vi "nii_head.vi"(8 "error in (no error)":errorcluster, 11 "file (use dialog)":path) -> (0 "error out":errorcluster, 3 "Data":T1 {"slice orientation" items=["transverse unflipped", "coronal unflipped", "sagittal unflipped", "transverse flipped", "coronal flipped", "sagittal flipped"]}, 4 "non-flip":bool, 5 "head":u8[](array[numeric]) format="%.0x")   [LabVIEW 2014]
uses:
  control/head_data.ctl
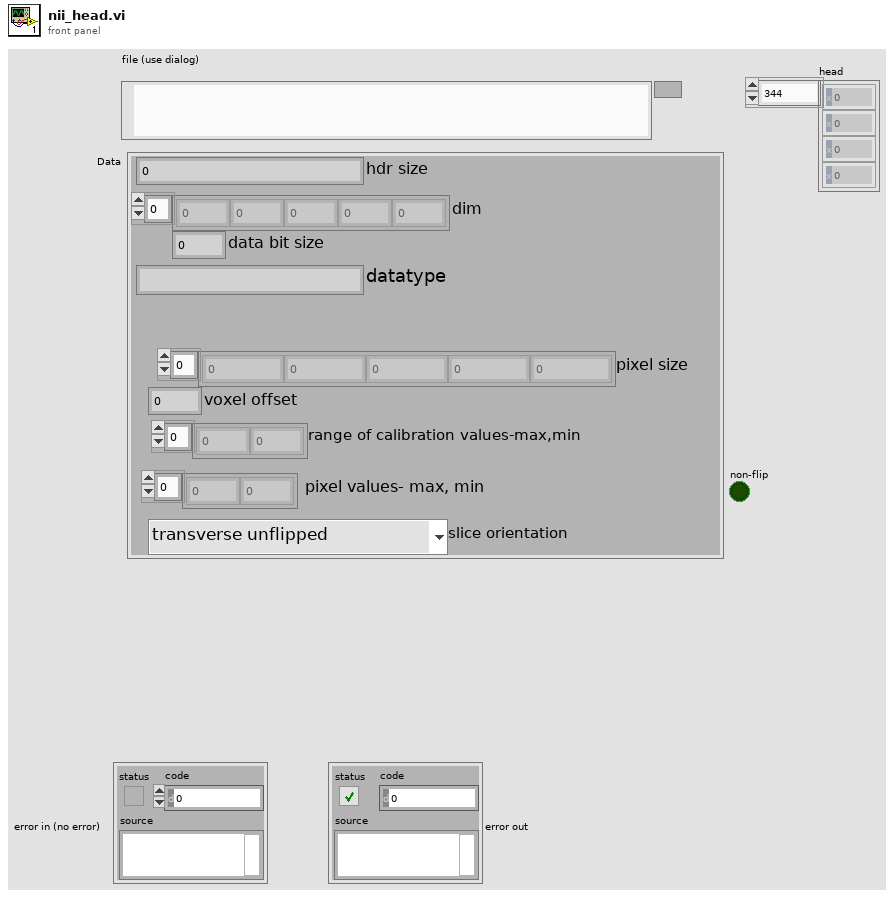
[diagram p1: front panel]
types:
  T1 = typedef "head_data.ctl" = cluster{"hdr size":i32, "dim":i32[], "data bit size":i32, "datatype":string, "pixel size ":sgl[], "voxel offset":sgl, "range of calibration values-max,min":sgl[], " pixel values- max, min":sgl[], "slice orientation":u16}
  T2 = enum16{"u_int8", "int8", "u_int16", "int16", "u_int32", "int32", "u_int64", "int64", "float", "double"}
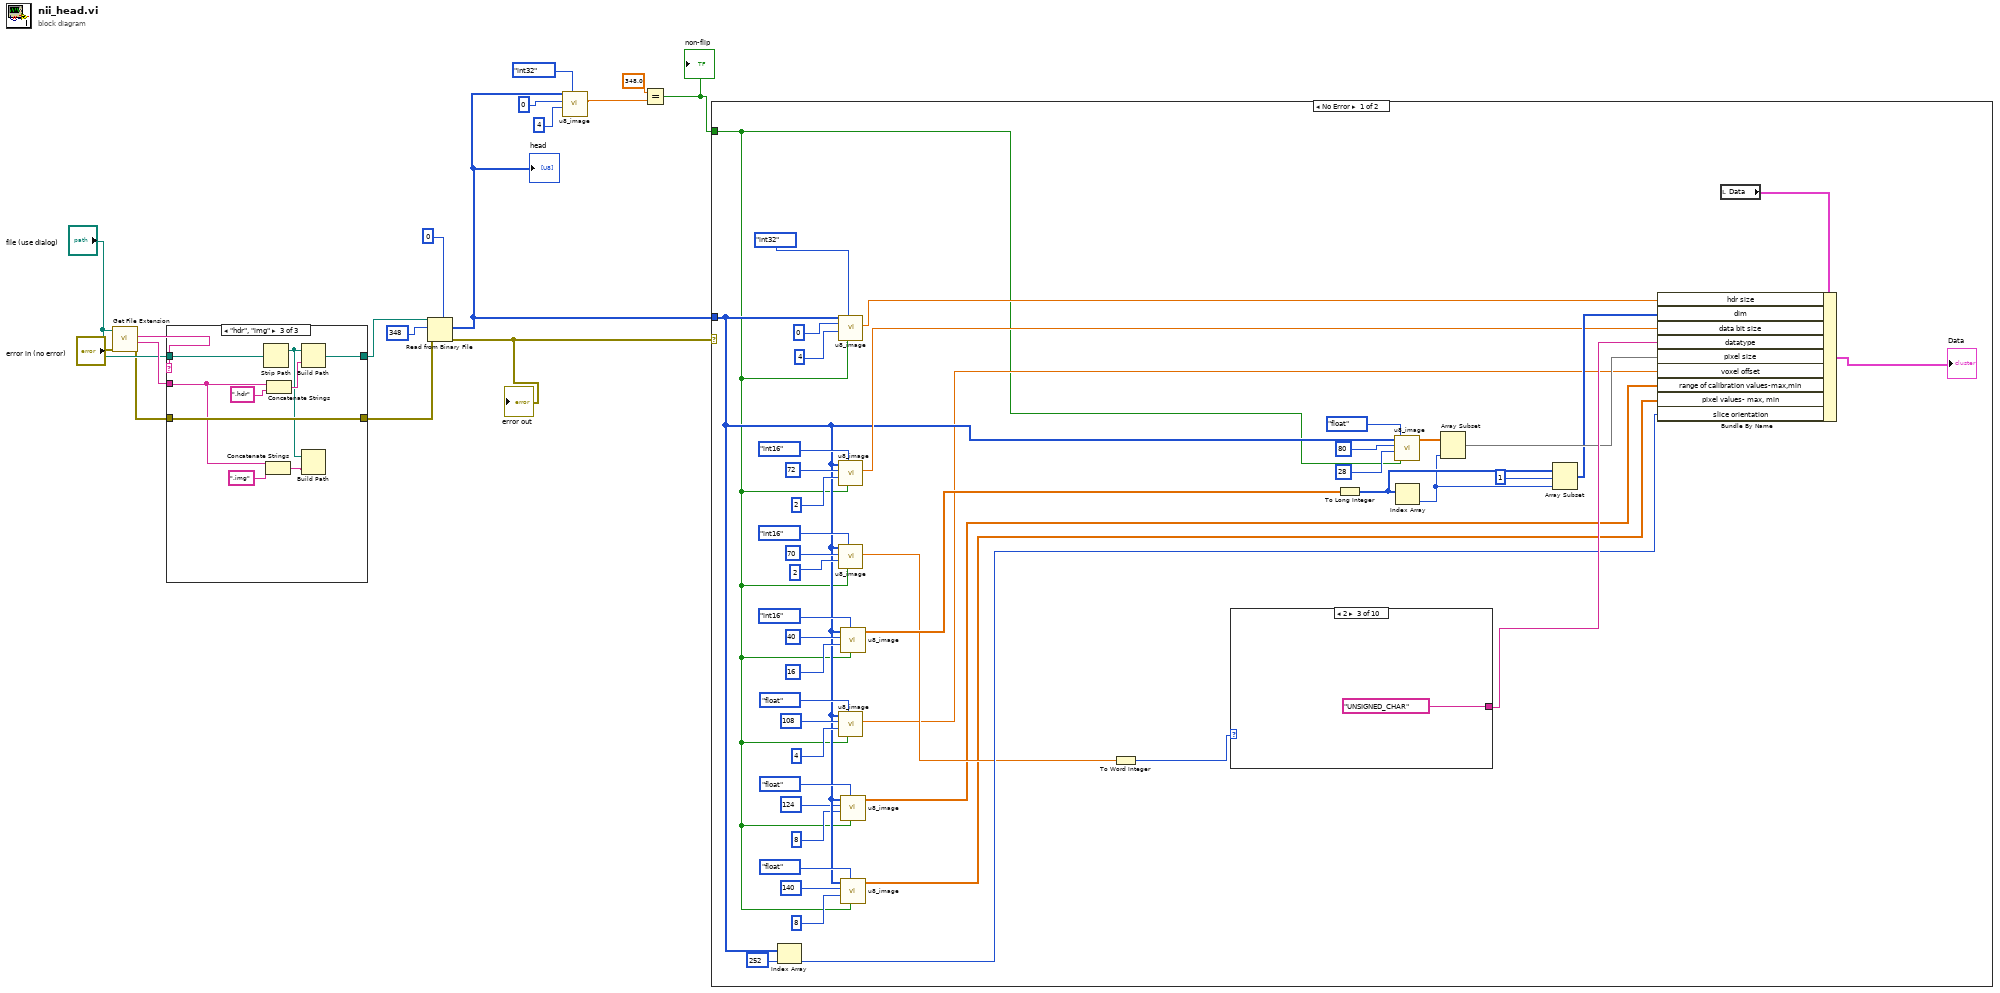
[diagram p0: block diagram]
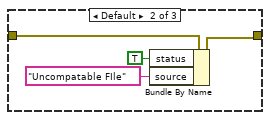
[diagram p3: hidden frame]
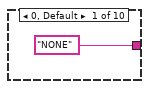
[diagram p4: hidden frame]
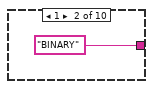
[diagram p5: hidden frame]
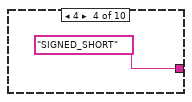
[diagram p6: hidden frame]
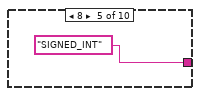
[diagram p7: hidden frame]
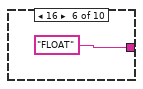
[diagram p8: hidden frame]
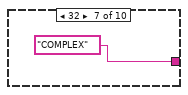
[diagram p9: hidden frame]
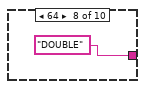
[diagram p10: hidden frame]
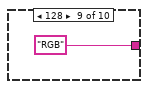
[diagram p11: hidden frame]
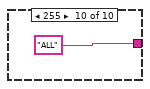
[diagram p12: hidden frame]
diagram:
  n1 = call <vilib>:"Get File Extension.vi"("error in (no error)"="error in (no error)", "file"="file (use dialog)") -> ("error out"=w13:errorcluster, "filename without extension"=w16:string, "lowercase file extension"=w17:string)  [unwired: 6 in, 1 out]
  n2 = case shown="\"hdr\", \"img\"" w17 {
    tunnel: "file (use dialog)" -> [w18 _ w28]
    tunnel: [w18 _ w30] -> w10
    tunnel: w16 -> [_ _ w24]
    tunnel: [w19 w22 w29] -> w14
    tunnel: w13 -> [w19 w23 w29]
    frame "nii" {
    }
    frame Default {
      n3 = Bundle By Name(cluster=w23, "status"=TRUE, "source"="Uncompatable FIle") -> (w22:errorcluster)
    }
    frame "hdr", "img" {
      n4 = Strip Path(path=w28) -> (stripped path=w27:path)  [unwired: 1 out]
      n5 = Concatenate Strings(w24, ".img" ("string")) -> (w26:string)
      n6 = Concatenate Strings(w24, ".hdr" ("string")) -> (w31:string)
      n7 = Build Path(base path=w27, name or relative path=w31) -> (appended path=w30:path)
      n8 = Build Path(base path=w27, name or relative path=w26) -> ()  [unwired: 1 out]
    }
  }
  n9 = Read from Binary File(5:u8 0, 8:w14, 10:348 ("count (1)"), 11:w10) -> (0:w9:errorcluster, 2:w5:u8[])  [unwired: 2 in, 2 out]
  "error out" <- w9
  "head" <- w5
  n10 = call "u8_image.vi"("Enum"=T2."int32", "length"=4, "index"=0, "array"=w5) -> ("Numeric"=w3:dbl)  [unwired: 6 in, 1 out]
  n11 = Equal?(x=348.0, y=w3) -> (x = y?=w6:bool)
  "non-flip" <- w6
  n12 = case shown="No Error" w9 {
    tunnel: w5 -> [w39 _]
    tunnel: w6 -> [w35 _]
    frame No Error {
      n13 = Index Array(array=w39, index=252) -> (element=w73:u8)
      n14 = call "u8_image.vi"("non-flip"=w35, "Enum"=T2."int32", "length"=4, "index"=0, "array"=w39) -> ("Numeric"=w67:dbl)  [unwired: 5 in, 1 out]
      n15 = call "u8_image.vi"("non-flip"=w35, "Enum"=T2."int16", "length"=2, "index"=72, "array"=w39) -> ("Numeric"=w58:dbl)  [unwired: 5 in, 1 out]
      n16 = call "u8_image.vi"("non-flip"=w35, "Enum"=T2."int16", "length"=2, "index"=70, "array"=w39) -> ("Numeric"=w54:dbl)  [unwired: 5 in, 1 out]
      n17 = call "u8_image.vi"("non-flip"=w35, "Enum"=T2."float", "length"=4, "index"=108, "array"=w39) -> ("Numeric"=w36:dbl)  [unwired: 5 in, 1 out]
      n18 = call "u8_image.vi"("non-flip"=w35, "Enum"=T2."int16", "length"=16, "index"=40, "array"=w39) -> ("Array"=w64:dbl[])  [unwired: 5 in, 1 out]
      n19 = call "u8_image.vi"("non-flip"=w35, "Enum"=T2."float", "length"=8, "index"=124, "array"=w39) -> ("Array"=w40:dbl[])  [unwired: 5 in, 1 out]
      n20 = call "u8_image.vi"("non-flip"=w35, "Enum"=T2."float", "length"=8, "index"=140, "array"=w39) -> ("Array"=w43:dbl[])  [unwired: 5 in, 1 out]
      n21 = To Word Integer(number=w54) -> (16bit integer=w53:i16)
      n22 = case shown="2" w53 {
        tunnel: ["NONE" "BINARY" "UNSIGNED_CHAR" "SIGNED_SHORT" "SIGNED_INT" "FLOAT" "COMPLEX" "DOUBLE" "RGB" "ALL"] -> w77
        frame 0, Default {
        }
        frame 1 {
        }
        frame 2 {
        }
        frame 4 {
        }
        frame 8 {
        }
        frame 16 {
        }
        frame 32 {
        }
        frame 64 {
        }
        frame 128 {
        }
        frame 255 {
        }
      }
      n23 = To Long Integer(number=w64) -> (32bit integer=w70:i32[])
      n24 = call "u8_image.vi"("non-flip"=w35, "Enum"=T2."float", "length"=28, "index"=80, "array"=w39) -> ("Array"=w50:dbl[])  [unwired: 5 in, 1 out]
      n25 = Index Array(array=w70) -> (element=w34:i32)  [unwired: 1 in]
      n26 = Array Subset(array=w50, length=w34) -> (w76:dbl[])  [unwired: 1 in]
      n27 = Array Subset(array=w70, index=1, length=w34) -> (w71:i32[])
      n28 = local read "Data"() -> (w75:T1)
      n29 = Bundle By Name(cluster=w75, "hdr size"=w67, "dim"=w71, "data bit size"=w58, "datatype"=w77, "pixel size"=w76, "voxel offset"=w36, "range of calibration values-max,min"=w40, "pixel values- max, min"=w43, "slice orientation"=w73) -> (→"Data":T1)
    }
    frame Error {
    }
  }
